vi "Write Indicator.vi"(5 "High Address":u32 format="%08x", 7 "Base Address":u32 format="%08x", 9 "Data":u32 format="%08x", 11 "Address":u32 format="%08x") -> (0 "Error?":bool, 2 "Offset":u32)   [LabVIEW 2011]
uses:
  uBlaze VIVM Globals.vi
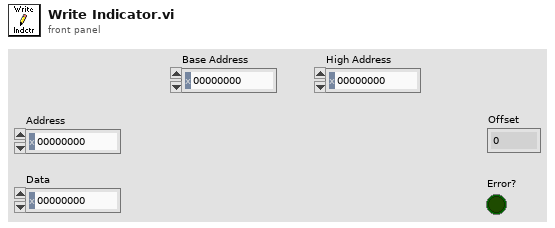
[diagram p1: front panel]
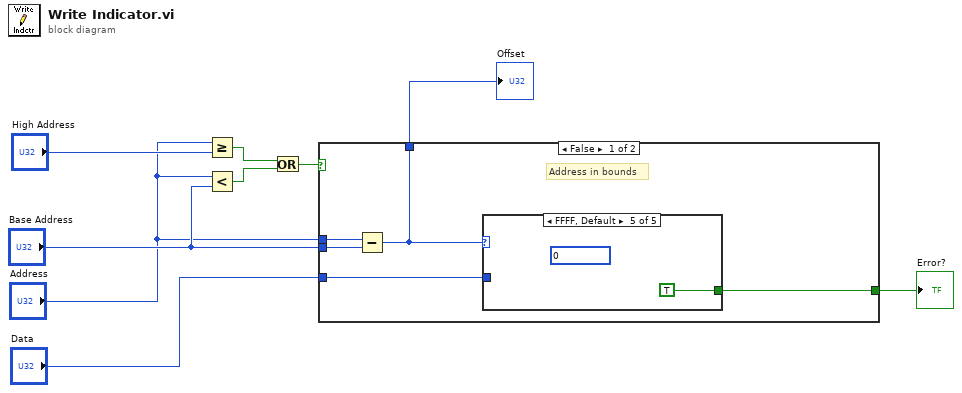
[diagram p0: block diagram]
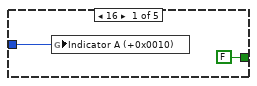
[diagram p2: hidden frame]
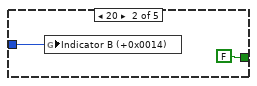
[diagram p3: hidden frame]
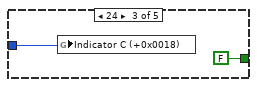
[diagram p4: hidden frame]
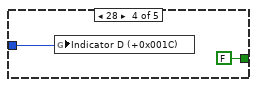
[diagram p5: hidden frame]
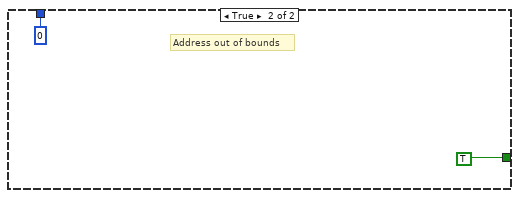
[diagram p6: hidden frame]
diagram:
  n1 = Greater Or Equal?(x="Address", y="High Address") -> (x >= y?=w3:bool)
  n2 = Less?(x="Address", y="Base Address") -> (x < y?=w2:bool)
  n3 = Or(x=w3, y=w2) -> (x .or. y?=w9:bool)
  n4 = case shown="False" w9 {
    tunnel: [w14 TRUE ("Error")] -> w8
    tunnel: "Data" -> [w13 _]
    tunnel: [w12 u32 0] -> w6
    tunnel: "Base Address" -> [w10 _]
    tunnel: "Address" -> [w11 _]
    frame False {
      # "Address in bounds"
      n5 = Subtract(x=w11, y=w10) -> (x-y=w12:u32)
      n6 = case shown="FFFF, Default" w12 {
        tunnel: [FALSE ("Error") FALSE ("Error") FALSE ("Error") FALSE ("Error") TRUE ("Error")] -> w14
        tunnel: w13 -> [w15 w17 w19 w21 _]
        frame 16 {
          n7 = global write "uBlaze VIVM Globals.vi" "Indicator A (+0x0010)"(w15) -> ()
        }
        frame 20 {
          n8 = global write "uBlaze VIVM Globals.vi" "Indicator B (+0x0014)"(w17) -> ()
        }
        frame 24 {
          n9 = global write "uBlaze VIVM Globals.vi" "Indicator C (+0x0018)"(w19) -> ()
        }
        frame 28 {
          n10 = global write "uBlaze VIVM Globals.vi" "Indicator D (+0x001C)"(w21) -> ()
        }
        frame 65535, Default {
          (unwired) 0 ("Data")
        }
      }
    }
    frame True {
      # "Address out of bounds"
    }
  }
  "Error?" <- w8
  "Offset" <- w6
